vi "test.vi"() -> ()   [LabVIEW 2010]
panel:
  out "cos(x)":dbl[](array[numeric])
  out "sin(x)":dbl[](array[numeric])
  out "subarray":dbl[](array[numeric])
  in  "Angle Array":dbl[](array[numeric])
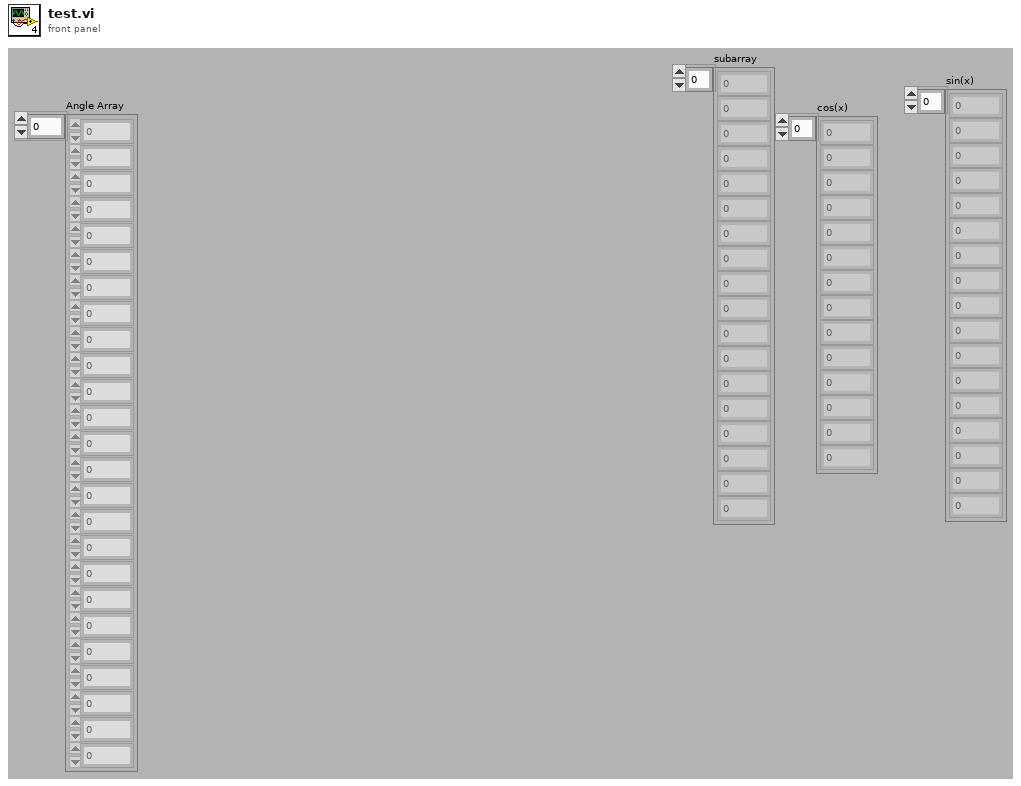
[diagram p1: front panel]
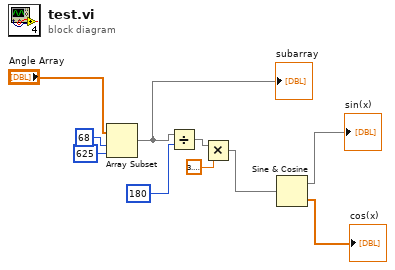
[diagram p0: block diagram]
diagram:
  n1 = Array Subset(array="Angle Array", index=68 ("length"), length=625) -> (w1:dbl[])
  "subarray" <- w1
  n2 = Divide(x=w1, y=180 ("length")) -> (x/y=w6:dbl[])
  n3 = Multiply(x=w6, y=3.141592653589793) -> (x*y=w4:dbl[])
  n4 = Sine & Cosine(0:w4) -> (1:→"sin(x)":dbl[], 2:→"cos(x)":dbl[])
